vi "Autonomous Independent.vi"() -> ()   [LabVIEW 2016]
doc: "This VI is called when autonomous begins, and will automatically be terminated when autonomous ends. You can carry out timed or sensor driven robot movement independently without needing to return to the caller."
uses:
  <vilib>/Rock Robotics/WPI/Solenoid/WPI_SolenoidValue.ctl
  <vilib>/Rock Robotics/WPI/Utilities/WPI_GetSetVariantRefNum.vi
  <vilib>/Rock Robotics/Network Tables/NT Write Numeric Array.vi
  <vilib>/Rock Robotics/Network Tables/NT Read String.vi
  <vilib>/Rock Robotics/WPI/RobotDrive/WPI_RobotDriveArcadeDrive_Standard(NoSaturation).vi
  <vilib>/Rock Robotics/WPI/Solenoid/WPI_SolenoidSetEnum.vi
panel:
  out "encodervalue 2":dbl
  out "Current Movement, for debugging":T1 {"Y Joystick Value" scale=1.0..-1.0; "X Joystick Value" scale=-1.0..1.0}
  in  "Array of robot movements":T2(array[cluster])=[{"X Joystick Value"=0.39393939393939403, "Y Joystick Value"=0.0, "Delay (sec)"=1.0, "Movement Name"="turn"}, {"X Joystick Value"=-0.3737373737373737, "Y Joystick Value"=0.0, "Delay (sec)"=1.0, "Movement Name"="turn back"}] {"Y Joystick Value" scale=1.0..-1.0; "X Joystick Value" scale=-1.0..1.0}
  out "encodervalue":dbl
  # "Be sure to right-click and choose Data Operations>>Make Current Value default if you want to save the array values with the VI"
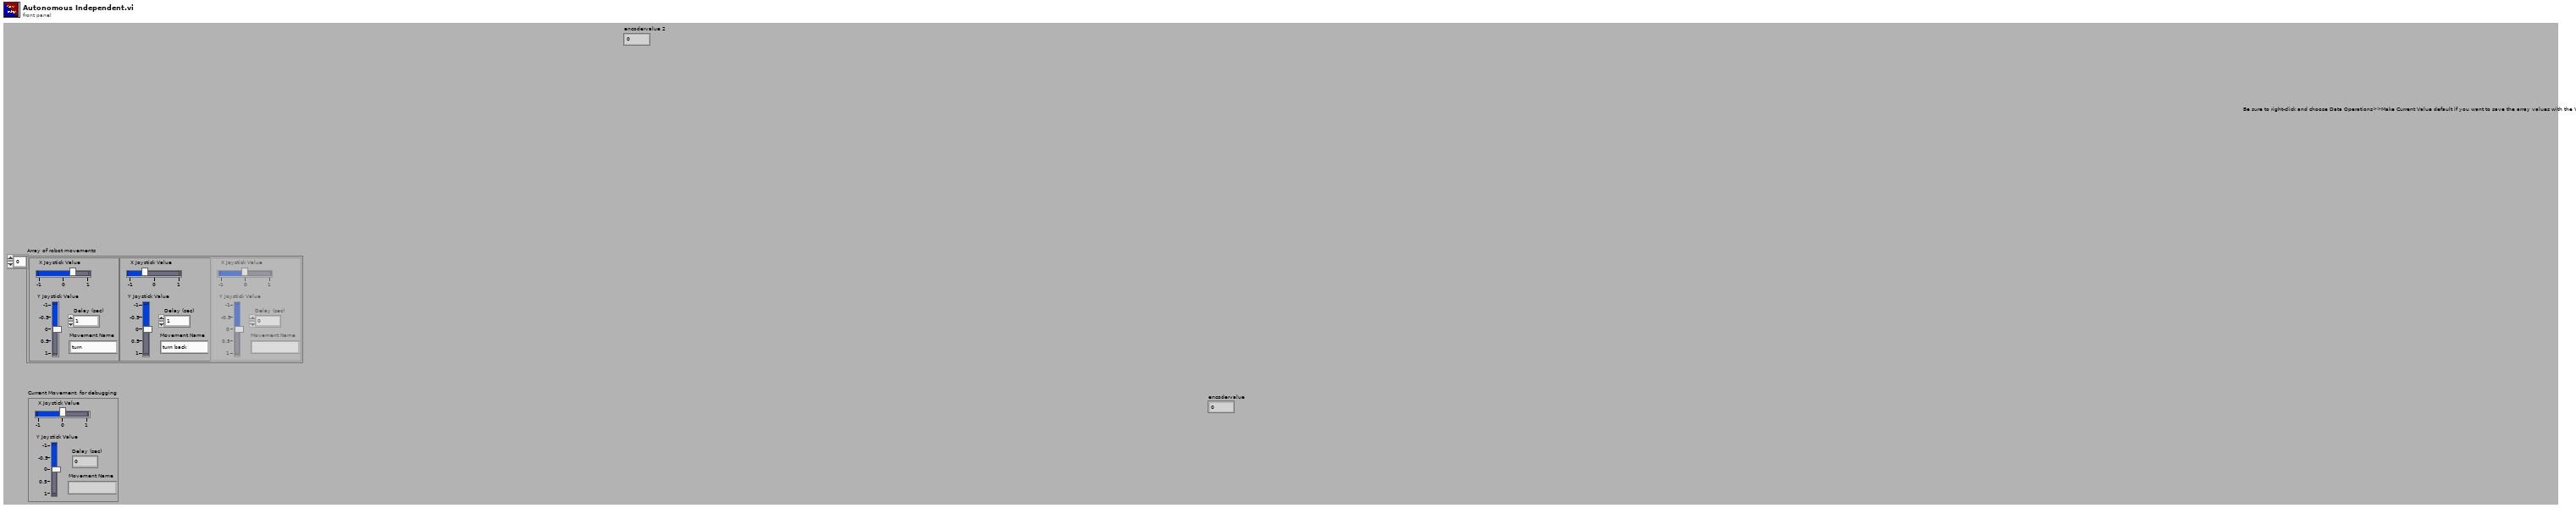
[diagram p1: front panel]
types:
  T1 = cluster{"X Joystick Value":dbl, "Y Joystick Value":dbl, "Delay (sec)":dbl, "Movement Name":string}
  T2 = cluster{"X Joystick Value":dbl, "Y Joystick Value":dbl, "Delay (sec)":dbl, "Movement Name":string}[]
  T3 = typedef "WPI_JoystickDevRef.ctl" = cluster{"Device":T4}
  T4 = typedef "WPI_JoystickDeviceEnum.ctl" = enum16{"USB 0", "USB 1", "USB 2", "USB 3", "USB 4", "USB 5"}
  T5 = typedef "WPI_EncoderDevRef.ctl" = cluster{"DevStatus":errorcluster, "EncoderIndex":T6, "CounterIndex":T7, "DistancePerCount":dbl, "Decoding Type":T8}
  T6 = typedef "FPGA_EncoderIdx.ctl" = enum8{"Enc 0", "Enc 1", "Enc 2", "Enc 3", "Enc 4", "Enc 5", "Enc 6", "Enc 7", "Invalid"}
  T7 = typedef "FPGA_CounterCtrSystemIndex.ctl" = enum8{"Ctr 0", "Ctr 1", "Ctr 2", "Ctr 3", "Ctr 4", "Ctr 5", "Ctr 6", "Ctr 7", "Invalid"}
  T8 = typedef "WPI_EncoderType.ctl" = enum16{"1x", "2x", "4x"}
  T9 = typedef "WPI_GyroDevRef.ctl" = cluster{"DevStatus":errorcluster, "Analog Channel":T10, "Offset":dbl, "Gain (VoltsPerDegree/Second)":dbl, "Gyro Type":enum16{"Analog", "XRS450"}, "Handle":i32, "SPI Bus":T11, "Device Found":bool, "Sample Rate":dbl, "Calibrate On Open":bool}
  T10 = typedef "FPGA_AIChannel.ctl" = enum8{"AI 0", "AI 1", "AI 2", "AI 3", "AI MXP 0", "AI MXP 1", "AI MXP 2", "AI MXP 3", "Invalid"}
  T11 = typedef "spi_bus.ctl" = enum16{"SPI On-Board, CS0", "SPI On-Board, CS1", "SPI On-Board, CS2", "SPI On-Board, CS3", "SPI MXP", "Invalid"}
  T12 = typedef "WPI_RobotDriveDevRef.ctl" = cluster{"DevStatus":errorcluster, "Motors[]":T13[], "Square Inputs":bool, "Max Output":dbl}
  T13 = typedef "WPI_MotorControlDeviceRef.ctl" = cluster{"DeviceStatus":errorcluster, "Type":T14, "PWM":cluster{"PWM Channel":T15, "DeadBand":T16}, "CAN":cluster{"Device Number":u8, "SetOutput VI Ref":variant, "GetOutput VI Ref":variant, "Enable VI Ref":variant, "Disable VI Ref":variant, "Data":variant}, "Invert":bool}
  T14 = typedef "WPI_MotorControlType.ctl" = enum16{"PWM", "CAN"}
  T15 = typedef "FPGA_DIOPWMChannel.ctl" = enum8{"PWM 0", "PWM 1", "PWM 2", "PWM 3", "PWM 4", "PWM 5", "PWM 6", "PWM 7", "PWM 8", "PWM 9", "PWM MXP 0", "PWM MXP 1", "PWM MXP 2", "PWM MXP 3", "PWM MXP 4", "PWM MXP 5", "PWM MXP 6", "PWM MXP 7", "PWM MXP 8", "PWM MXP 9", "Invalid"}
  T16 = typedef "WPI_PWMDeadband.ctl" = cluster{"Name":string, "maxPositivePwm":i32, "minPositivePwm":i32, "centerPwm":i32, "maxNegativePwm":i32, "minNegativePwm":i32, "angularRange":u16}
  T17 = typedef "WPI_SolenoidDevRef.ctl" = cluster{"DevStatus":errorcluster, "Pneumatics Control Module":u8, "Forward Solenoid Channel":T18, "Reverse Solenoid Channel":T18}
  T18 = typedef "WPI_SolenoidChannel.ctl" = enum8{"Solenoid 0", "Solenoid 1", "Solenoid 2", "Solenoid 3", "Solenoid 4", "Solenoid 5", "Solenoid 6", "Solenoid 7", "Invalid"}
  T19 = typedef "WPI_SolenoidValue.ctl" = enum16{"Off", "On", "Forward", "Reverse"}
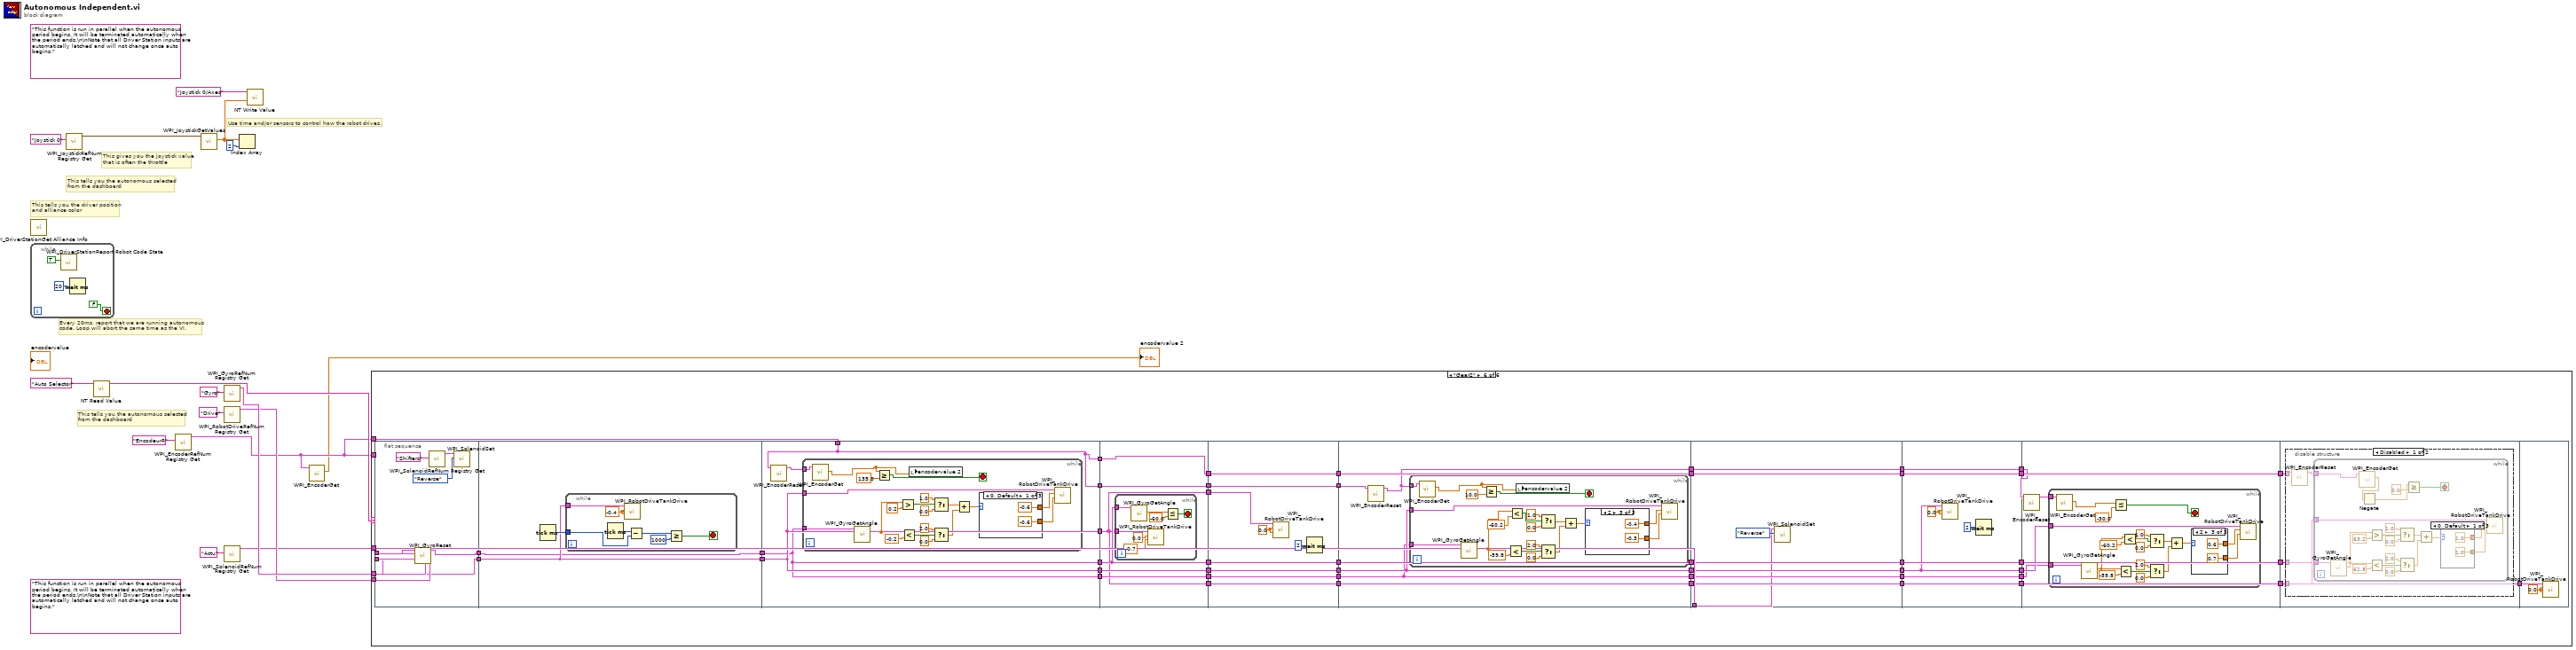
[diagram p0: block diagram]
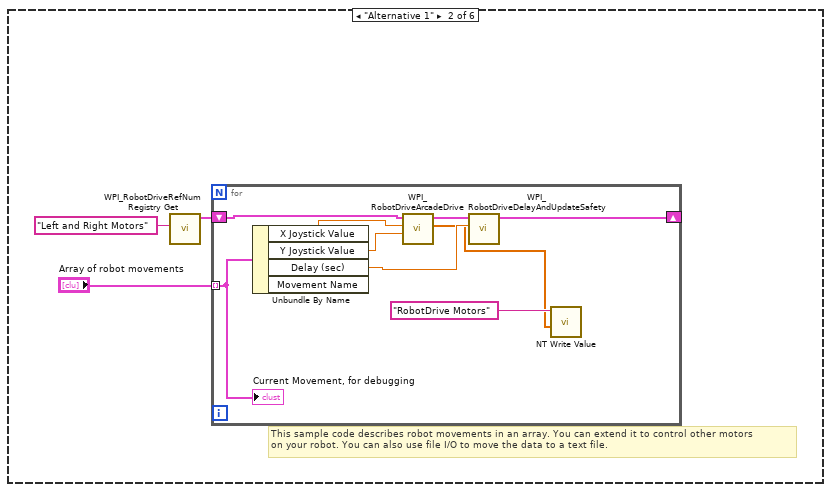
[diagram p3: hidden frame]
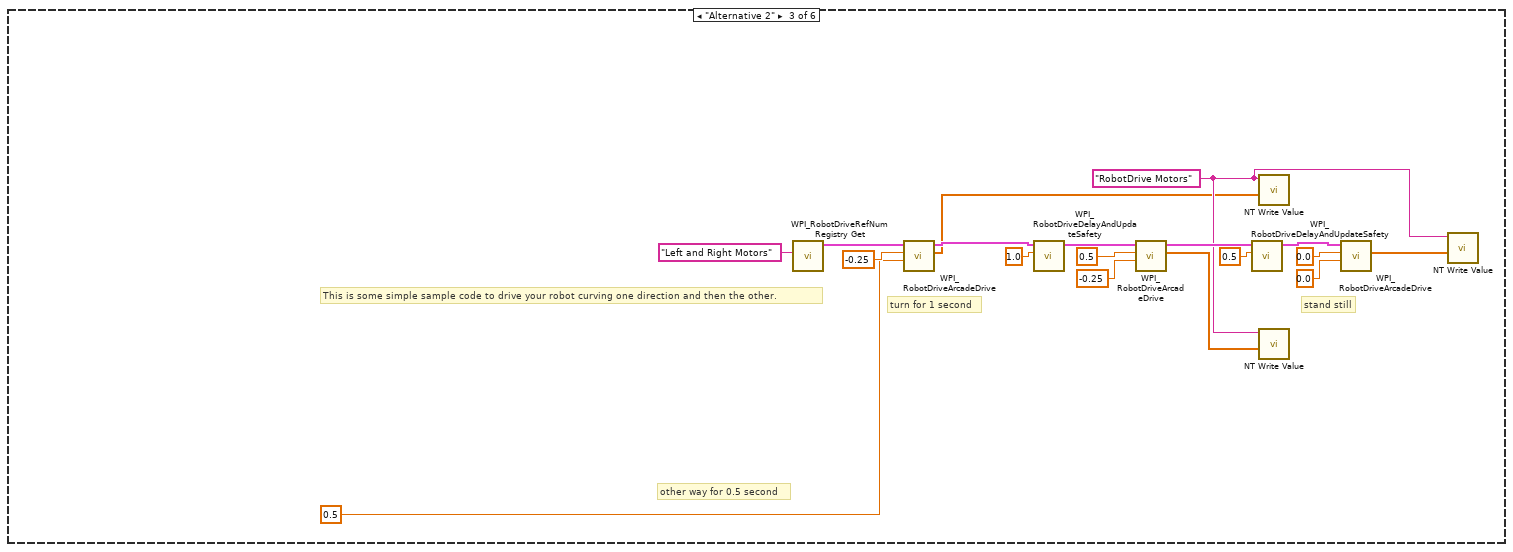
[diagram p4: hidden frame]
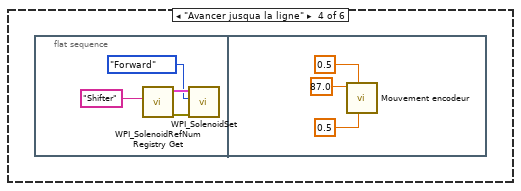
[diagram p5: hidden frame]
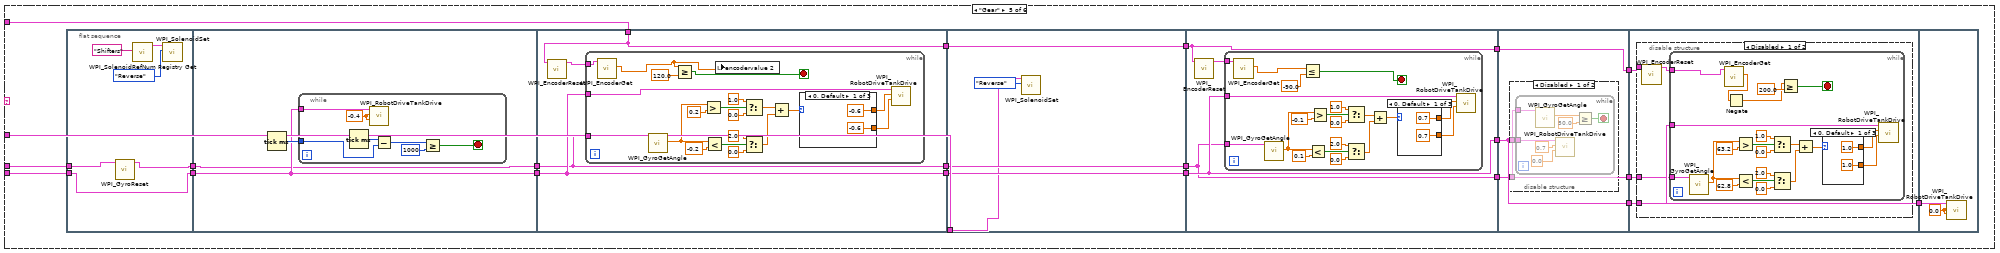
[diagram p6: hidden frame]
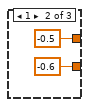
[diagram p7: hidden frame]
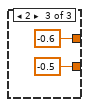
[diagram p8: hidden frame]
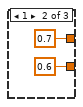
[diagram p9: hidden frame]
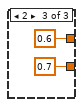
[diagram p10: hidden frame]
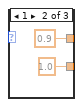
[diagram p12: hidden frame]
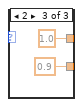
[diagram p13: hidden frame]
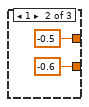
[diagram p15: hidden frame]
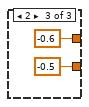
[diagram p16: hidden frame]
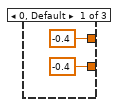
[diagram p17: hidden frame]
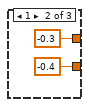
[diagram p18: hidden frame]
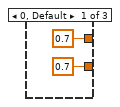
[diagram p19: hidden frame]
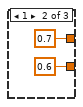
[diagram p20: hidden frame]
diagram:
  (unwired) "This function is run in parallel when the autonomous period begins. It will be terminated automatically when the period ends.\n\nNote that all Driver Station inputs are automatically latched and will not change once auto begins."
  (unwired) "This function is run in parallel when the autonomous period begins. It will be terminated automatically when the period ends.\n\nNote that all Driver Station inputs are automatically latched and will not change once auto begins."
  # "This tells you the autonomous selected\nfrom the dashboard"
  # "This tells you the autonomous selected\nfrom the dashboard"
  # "Every 20ms, report that we are running autonomous\ncode. Loop will abort the same time as the VI."
  # "This gives you the joystick value\nthat is often the throttle"
  # "Use time and/or sensors to control how the robot drives."
  # "This tells you the driver position\nand alliance color"
  n1 = call <vilib>:"WPI_DriverStationGet Alliance Info.vi"() -> ()  [unwired: 12 out]
  n2 = while {
    stop <- FALSE stop-if-true
    n3 = call <vilib>:"WPI_DriverStationReport Robot Code State.vi"("Autonomous"=TRUE) -> ()  [unwired: 10 in, 1 out]
    n4 = Wait (ms)(milliseconds to wait=u32 20) -> ()  [unwired: 1 out]
  }
  n5 = call <vilib>:"WPI_JoystickRefNum Registry Get.vi"("refnum name"="Joystick 0") -> ("JoystickDevRef"=w15:T3)  [unwired: 1 in, 9 out]
  n6 = call-poly <vilib>:"NT Read Value.vi"("Name"="Auto Selector") -> ("String"=w4:string)  [unwired: 9 in, 1 out]
  n7 = call <vilib>:"WPI_EncoderRefNum Registry Get.vi"("refnum name"="EncodeurR") -> ("EncoderDevRef"=w2:T5)  [unwired: 9 in, 1 out]
  n8 = call <vilib>:"WPI_JoystickGetValues.vi"("JoystickDevRef"=w15) -> ("Axes"=w13:dbl[])  [unwired: 6 in, 4 out]
  n9 = call <vilib>:"WPI_GyroRefNum Registry Get.vi"("refnum name"="Gyro") -> ("GyroDevRef"=w6:T9)  [unwired: 9 in, 1 out]
  n10 = call <vilib>:"WPI_RobotDriveRefNum Registry Get.vi"("refnum name"="Drive") -> ("RobotDriveDevRef"=w5:T12)  [unwired: 9 in, 1 out]
  n11 = call <vilib>:"WPI_SolenoidRefNum Registry Get.vi"("refnum name"="Actu") -> ("SolenoidDevRef"=w3:T17)  [unwired: 9 in, 1 out]
  n12 = Index Array(array=w13, index=2) -> ()  [unwired: 1 out]
  n13 = call-poly <vilib>:"NT Write Value.vi"("Numeric Array"=w13, "Name"="Joystick 0/Axes") -> ()  [unwired: 9 in, 1 out]
  n14 = call <vilib>:"WPI_EncoderGet.vi"("EncoderDevRef"=w2) -> ("Distance"=→"encodervalue 2":dbl)  [unwired: 5 in, 5 out]
  n15 = case shown="\"Gear2\"" w4 {
    tunnel: w5 -> [_ _ _ _ w77 w249]
    tunnel: w6 -> [_ _ _ _ w72 w250]
    tunnel: w2 -> [_ _ _ _ w66 _]
    tunnel: w2 -> [_ _ _ _ _ w248]
    tunnel: w3 -> [_ _ _ _ w57 w219]
    frame Default {
      # "You can put your main auto here, or you can right-click on the case and make any\nother frame be the default case."
      # "This is the frame that will execute if no selection is made, or if it is not recognized"
    }
    frame "Alternative 1" {
      # "This sample code describes robot movements in an array. You can extend it to control other motors\non your robot. You can also use file I/O to move the data to a text file."
      n16 = call <vilib>:"WPI_RobotDriveRefNum Registry Get.vi"("refnum name"="Left and Right Motors") -> ("RobotDriveDevRef"=w21:T12)  [unwired: 1 in, 9 out]
      n17 = for {
        shift-right: [w29] -> _
        shift-left: w21 -> [w30]
        tunnel: "Array of robot movements" -> [w25] mode=indexing
        n18 = Unbundle By Name(w25) -> ("X Joystick Value"=w28:dbl, "Y Joystick Value"=w27:dbl, "Delay (sec)"=w26:dbl)  [unwired: 1 out]
        n19 = call-poly <vilib>:"WPI_RobotDriveArcadeDrive.vi"("Y axis value"=w27, "X axis value"=w28, "RobotDriveDevRef"=w30) -> ("Motor Values"=w23:dbl[], "RobotDriveDevRef"=w31:T12)  [unwired: 1 in, 6 out]
        n20 = call <vilib>:"WPI_RobotDriveDelayAndUpdateSafety.vi"("Delay (s)"=w26, "RobotDriveDevRef"=w31) -> ("RobotDriveDevRef 2"=w29:T12)  [unwired: 8 in, 1 out]
        n21 = call-poly <vilib>:"NT Write Value.vi"("Numeric Array"=w23, "Name"="RobotDrive Motors") -> ()  [unwired: 9 in, 1 out]
        "Current Movement, for debugging" <- w25
      }
    }
    frame "Alternative 2" {
      w33 = "RobotDrive Motors" ("Name")
      # "This is some simple sample code to drive your robot curving one direction and then the other."
      # "stand still"
      # "other way for 0.5 second"
      # "turn for 1 second"
      n22 = call <vilib>:"WPI_RobotDriveRefNum Registry Get.vi"("refnum name"="Left and Right Motors") -> ("RobotDriveDevRef"=w49:T12)  [unwired: 1 in, 9 out]
      n23 = call-poly <vilib>:"WPI_RobotDriveArcadeDrive.vi"("Y axis value"=0.5 ("X axis value"), "X axis value"=-0.25, "RobotDriveDevRef"=w49) -> ("Motor Values"=w32:dbl[], "RobotDriveDevRef"=w42:T12)  [unwired: 1 in, 6 out]
      n24 = call <vilib>:"WPI_RobotDriveDelayAndUpdateSafety.vi"("Delay (s)"=1.0, "RobotDriveDevRef"=w42) -> ("RobotDriveDevRef 2"=w43:T12)  [unwired: 8 in, 1 out]
      n25 = call-poly <vilib>:"WPI_RobotDriveArcadeDrive.vi"("Y axis value"=-0.25 ("X axis value"), "X axis value"=0.5, "RobotDriveDevRef"=w43) -> ("Motor Values"=w34:dbl[], "RobotDriveDevRef"=w44:T12)  [unwired: 1 in, 6 out]
      n26 = call <vilib>:"WPI_RobotDriveDelayAndUpdateSafety.vi"("Delay (s)"=0.5, "RobotDriveDevRef"=w44) -> ("RobotDriveDevRef 2"=w45:T12)  [unwired: 8 in, 1 out]
      n27 = call-poly <vilib>:"NT Write Value.vi"("Numeric Array"=w32, "Name"=w33) -> ()  [unwired: 9 in, 1 out]
      n28 = call-poly <vilib>:"NT Write Value.vi"("Numeric Array"=w34, "Name"=w33) -> ()  [unwired: 9 in, 1 out]
      n29 = call-poly <vilib>:"WPI_RobotDriveArcadeDrive.vi"("Y axis value"=0.0 ("X axis value"), "X axis value"=0.0, "RobotDriveDevRef"=w45) -> ("Motor Values"=w35:dbl[])  [unwired: 1 in, 7 out]
      n30 = call-poly <vilib>:"NT Write Value.vi"("Numeric Array"=w35, "Name"=w33) -> ()  [unwired: 9 in, 1 out]
    }
    frame "Avancer jusqua la ligne" {
      n31 = flat-sequence {
        frame #0 {
          n32 = call <vilib>:"WPI_SolenoidRefNum Registry Get.vi"("refnum name"="Shifter") -> ("error out"=w52:errorcluster, "SolenoidDevRef"=w51:T17)  [unwired: 9 in]
          n33 = call-poly <vilib>:"WPI_SolenoidSet.vi"("error in (no error)"=w52, "Value"=WPI_SolenoidValue."Forward", "SolenoidDevRef"=w51) -> ()  [unwired: 7 in, 2 out]
        }
        frame #1 {
          n34 = call "Mouvement encodeur.vi"("Vitesse initiale"=0.5, "Temps acceleration"=0.5, "Distance"=87.0) -> ()  [unwired: 9 in]
        }
      }
    }
    frame "Gear" {
      n35 = flat-sequence {
        tunnel: [w79] -> w76
        tunnel: w77 -> [w79]
        tunnel: [w78] -> w73
        tunnel: w72 -> [w80]
        tunnel: w76 -> [w85]
        tunnel: [w85] -> w75
        tunnel: [w84] -> w74
        tunnel: w73 -> [w84]
        tunnel: w75 -> [w97]
        tunnel: [w97] -> w63
        tunnel: w74 -> [w96]
        tunnel: [w96] -> w61
        tunnel: w66 -> [w95]
        tunnel: [w95] -> w59
        tunnel: w63 -> [w128]
        tunnel: [w128] -> w62
        tunnel: w61 -> [w127]
        tunnel: [w127] -> w60
        tunnel: w59 -> [w126]
        tunnel: [w126] -> w58
        tunnel: w57 -> [w125]
        tunnel: w62 -> [w132]
        tunnel: [w132] -> w71
        tunnel: w60 -> [w131]
        tunnel: [w131] -> w70
        tunnel: w58 -> [w130]
        tunnel: [w130] -> w65
        tunnel: w71 -> [w161]
        tunnel: [w161] -> w69
        tunnel: w70 -> [w160]
        tunnel: [w160] -> w67
        tunnel: w65 -> [w159]
        tunnel: [w159] -> w64
        tunnel: w69 -> [w173]
        tunnel: [w173] -> w68
        tunnel: w67 -> [w172]
        tunnel: w64 -> [w171]
        tunnel: w68 -> [w205]
        frame #0 {
          n36 = call <vilib>:"WPI_GyroReset.vi"("GyroDevRef"=w80) -> ("GyroDevRef"=w78:T9)  [unwired: 9 in, 1 out]
          n37 = call <vilib>:"WPI_SolenoidRefNum Registry Get.vi"("refnum name"="Shifters") -> ("SolenoidDevRef"=w83:T17)  [unwired: 9 in, 1 out]
          n38 = call-poly <vilib>:"WPI_SolenoidSet.vi"("Value"=WPI_SolenoidValue."Reverse", "SolenoidDevRef"=w83) -> ()  [unwired: 8 in, 2 out]
        }
        frame #1 {
          n39 = Tick Count (ms)() -> (millisecond timer value=w86:u32)
          n40 = while {
            tunnel: w85 -> [w92]
            tunnel: w86 -> [w90]
            stop <- w87 stop-if-true
            w93 = -0.4 ("Left axis value")
            n41 = Tick Count (ms)() -> (millisecond timer value=w91:u32)
            n42 = call <vilib>:"WPI_RobotDriveTankDrive.vi"("Right axis value"=w93, "Left axis value"=w93, "RobotDriveDevRef"=w92) -> ()  [unwired: 6 in, 3 out]
            n43 = Subtract(x=w91, y=w90) -> (x-y=w89:u32)
            n44 = Greater Or Equal?(x=w89, y=u32 1000) -> (x >= y?=w87:bool)
          }
        }
        frame #2 {
          n45 = call <vilib>:"WPI_EncoderReset.vi"("EncoderDevRef"=w95) -> ("EncoderDevRef"=w94:T5)  [unwired: 9 in, 1 out]
          n46 = while {
            tunnel: w97 -> [w117]
            tunnel: w96 -> [w116]
            tunnel: w94 -> [w99]
            stop <- w100 stop-if-true
            n47 = call <vilib>:"WPI_EncoderGet.vi"("EncoderDevRef"=w99) -> ("Distance"=w98:dbl)  [unwired: 5 in, 5 out]
            n48 = call <vilib>:"WPI_GyroGetAngle.vi"("GyroDevRef"=w116) -> ("Angle"=w103:dbl)  [unwired: 6 in, 4 out]
            n49 = Greater Or Equal?(x=w98, y=120.0) -> (x >= y?=w100:bool)
            n50 = Greater?(x=w103, y=0.2) -> (0:w114:bool)
            n51 = Less?(x=w103, y=-0.2) -> (x < y?=w102:bool)
            n52 = local write "encodervalue 2"(w98) -> ()
            n53 = Select(t=1.0, s=w114, f=0.0) -> (s? t:f=w109:dbl)
            n54 = Select(t=2.0, s=w102, f=0.0) -> (s? t:f=w108:dbl)
            n55 = Add(x=w109, y=w108) -> (x+y=w107:dbl)
            n56 = case shown="0, Default" w107 {
              tunnel: [-0.6 ("t") -0.5 ("t") -0.6 ("t")] -> w106
              tunnel: [-0.6 ("f") -0.6 ("f") -0.5 ("f")] -> w105
              frame 0, Default {
              }
              frame 1 {
              }
              frame 2 {
              }
            }
            n57 = call <vilib>:"WPI_RobotDriveTankDrive.vi"("Right axis value"=w105, "Left axis value"=w106, "RobotDriveDevRef"=w117) -> ()  [unwired: 6 in, 3 out]
          }
        }
        frame #3 {
          n58 = call-poly <vilib>:"WPI_SolenoidSet.vi"("Value"=WPI_SolenoidValue."Reverse", "SolenoidDevRef"=w125) -> ()  [unwired: 8 in, 2 out]
        }
        frame #4 {
          n59 = call <vilib>:"WPI_EncoderReset.vi"("EncoderDevRef"=w130) -> ("EncoderDevRef"=w129:T5)  [unwired: 9 in, 1 out]
          n60 = while {
            tunnel: w132 -> [w140]
            tunnel: w131 -> [w137]
            tunnel: w129 -> [w134]
            stop <- w135 stop-if-true
            n61 = call <vilib>:"WPI_EncoderGet.vi"("EncoderDevRef"=w134) -> ("Distance"=w133:dbl)  [unwired: 5 in, 5 out]
            n62 = call <vilib>:"WPI_GyroGetAngle.vi"("GyroDevRef"=w137) -> ("Angle"=w151:dbl)  [unwired: 6 in, 4 out]
            n63 = Less Or Equal?(x=w133, y=-90.0) -> (x <= y?=w135:bool)
            n64 = Less?(x=w151, y=0.1) -> (x < y?=w152:bool)
            n65 = Greater?(x=w151, y=-0.1) -> (0:w142:bool)
            n66 = Select(t=1.0, s=w142, f=0.0) -> (s? t:f=w147:dbl)
            n67 = Select(t=2.0, s=w152, f=0.0) -> (s? t:f=w148:dbl)
            n68 = Add(x=w147, y=w148) -> (x+y=w149:dbl)
            n69 = case shown="0, Default" w149 {
              tunnel: [0.7 ("t") 0.7 ("t") 0.6 ("t")] -> w139
              tunnel: [0.7 ("f") 0.6 ("f") 0.7 ("f")] -> w138
              frame 0, Default {
              }
              frame 1 {
              }
              frame 2 {
              }
            }
            n70 = call <vilib>:"WPI_RobotDriveTankDrive.vi"("Right axis value"=w138, "Left axis value"=w139, "RobotDriveDevRef"=w140) -> ()  [unwired: 6 in, 3 out]
          }
        }
        frame #5 {
          n71 = disable-structure shown="Disabled" {
            disable-tunnel: w161 -> [w163 _]
            disable-tunnel: w160 -> [w162 _]
            frame Disabled {
              n72 = while {
                tunnel: w162 -> [w167]
                tunnel: w163 -> [w164]
                stop <- w168 stop-if-true
                n73 = call <vilib>:"WPI_GyroGetAngle.vi"("GyroDevRef"=w167) -> ("Angle"=w170:dbl)  [unwired: 6 in, 4 out]
                n74 = call <vilib>:"WPI_RobotDriveTankDrive.vi"("Right axis value"=0.0, "Left axis value"=0.7, "RobotDriveDevRef"=w164) -> ()  [unwired: 6 in, 3 out]
                n75 = Greater Or Equal?(x=w170, y=50.0) -> (x >= y?=w168:bool)
              }
            }
            frame Enabled {
            }
          }
        }
        frame #6 {
          n76 = disable-structure shown="Disabled" {
            disable-tunnel: w173 -> [w177 _]
            disable-tunnel: w172 -> [w176 _]
            disable-tunnel: w171 -> [w175 _]
            frame Disabled {
              n77 = call <vilib>:"WPI_EncoderReset.vi"("EncoderDevRef"=w175) -> ("EncoderDevRef"=w174:T5)  [unwired: 9 in, 1 out]
              n78 = while {
                tunnel: w177 -> [w198]
                tunnel: w176 -> [w196]
                tunnel: w174 -> [w180]
                stop <- w197 stop-if-true
                n79 = call <vilib>:"WPI_GyroGetAngle.vi"("GyroDevRef"=w196) -> ("Angle"=w183:dbl)  [unwired: 6 in, 4 out]
                n80 = call <vilib>:"WPI_EncoderGet.vi"("EncoderDevRef"=w180) -> ("Distance"=w179:dbl)  [unwired: 5 in, 5 out]
                n81 = Negate(x=w179) -> (-x=w178:dbl)
                n82 = Greater?(x=w183, y=63.2) -> (0:w194:bool)
                n83 = Less?(x=w183, y=62.8) -> (x < y?=w182:bool)
                n84 = Select(t=1.0, s=w194, f=0.0) -> (s? t:f=w189:dbl)
                n85 = Select(t=2.0, s=w182, f=0.0) -> (s? t:f=w188:dbl)
                n86 = Greater Or Equal?(x=w178, y=200.0) -> (x >= y?=w197:bool)
                n87 = Add(x=w189, y=w188) -> (x+y=w187:dbl)
                n88 = case shown="0, Default" w187 {
                  tunnel: [1.0 ("t") 0.9 ("t") 1.0 ("t")] -> w186
                  tunnel: [1.0 ("f") 1.0 ("f") 0.9 ("f")] -> w185
                  frame 0, Default {
                  }
                  frame 1 {
                  }
                  frame 2 {
                  }
                }
                n89 = call <vilib>:"WPI_RobotDriveTankDrive.vi"("Right axis value"=w185, "Left axis value"=w186, "RobotDriveDevRef"=w198) -> ()  [unwired: 6 in, 3 out]
              }
            }
            frame Enabled {
            }
          }
        }
        frame #7 {
          w206 = 0.0 ("Left axis value")
          n90 = call <vilib>:"WPI_RobotDriveTankDrive.vi"("Right axis value"=w206, "Left axis value"=w206, "RobotDriveDevRef"=w205) -> ()  [unwired: 6 in, 3 out]
        }
      }
    }
    frame "Gear2" {
      n91 = flat-sequence {
        tunnel: [w257] -> w255
        tunnel: w249 -> [w257]
        tunnel: [w256] -> w254
        tunnel: w250 -> [w258]
        tunnel: w255 -> [w263]
        tunnel: [w263] -> w253
        tunnel: [w262] -> w252
        tunnel: w254 -> [w262]
        tunnel: w253 -> [w274]
        tunnel: [w274] -> w247
        tunnel: w252 -> [w273]
        tunnel: [w273] -> w246
        tunnel: w248 -> [w272]
        tunnel: [w272] -> w245
        tunnel: [w274] -> w244
        tunnel: [w273] -> w243
        tunnel: [w272] -> w242
        tunnel: w247 -> [w302]
        tunnel: [w302] -> w238
        tunnel: w246 -> [w307]
        tunnel: [w307] -> w236
        tunnel: [w306] -> w234
        tunnel: w245 -> [w306]
        tunnel: [w305] -> w232
        tunnel: w244 -> [w305]
        tunnel: [w304] -> w230
        tunnel: w243 -> [w304]
        tunnel: [w303] -> w228
        tunnel: w242 -> [w303]
        tunnel: [w302] -> w226
        tunnel: w238 -> [w323]
        tunnel: [w323] -> w237
        tunnel: w236 -> [w322]
        tunnel: [w322] -> w235
        tunnel: w234 -> [w321]
        tunnel: [w321] -> w233
        tunnel: w232 -> [w320]
        tunnel: [w320] -> w231
        tunnel: w230 -> [w319]
        tunnel: [w319] -> w229
        tunnel: w228 -> [w318]
        tunnel: [w318] -> w227
        tunnel: w226 -> [w316]
        tunnel: w237 -> [w330]
        tunnel: [w330] -> w225
        tunnel: w235 -> [w329]
        tunnel: [w329] -> w224
        tunnel: w233 -> [w328]
        tunnel: [w328] -> w223
        tunnel: w231 -> [w327]
        tunnel: w229 -> [w326]
        tunnel: w227 -> [w324]
        tunnel: [w327] -> w222
        tunnel: [w326] -> w221
        tunnel: [w325] -> w220
        tunnel: w225 -> [w364]
        tunnel: [w364] -> w218
        tunnel: w224 -> [w363]
        tunnel: [w363] -> w216
        tunnel: w223 -> [w362]
        tunnel: [w362] -> w214
        tunnel: w222 -> [w361]
        tunnel: [w361] -> w212
        tunnel: w221 -> [w360]
        tunnel: [w360] -> w210
        tunnel: w220 -> [w359]
        tunnel: [w359] -> w208
        tunnel: w219 -> [w357]
        tunnel: w218 -> [w372]
        tunnel: [w372] -> w217
        tunnel: w216 -> [w371]
        tunnel: [w371] -> w215
        tunnel: w214 -> [w370]
        tunnel: [w370] -> w213
        tunnel: w212 -> [w365]
        tunnel: [w365] -> w211
        tunnel: w210 -> [w369]
        tunnel: [w369] -> w209
        tunnel: w208 -> [w368]
        tunnel: [w368] -> w207
        tunnel: w217 -> [w379]
        tunnel: [w379] -> w241
        tunnel: w215 -> [w378]
        tunnel: [w378] -> w240
        tunnel: w213 -> [w377]
        tunnel: [w377] -> w239
        tunnel: w211 -> [w375]
        tunnel: w209 -> [w374]
        tunnel: w207 -> [w373]
        tunnel: w241 -> [w408]
        tunnel: [w408] -> w251
        tunnel: w240 -> [w407]
        tunnel: w239 -> [w406]
        tunnel: w251 -> [w440]
        frame #0 {
          n92 = call <vilib>:"WPI_GyroReset.vi"("GyroDevRef"=w258) -> ("GyroDevRef"=w256:T9)  [unwired: 9 in, 1 out]
          n93 = call <vilib>:"WPI_SolenoidRefNum Registry Get.vi"("refnum name"="Shifters") -> ("SolenoidDevRef"=w261:T17)  [unwired: 9 in, 1 out]
          n94 = call-poly <vilib>:"WPI_SolenoidSet.vi"("Value"=WPI_SolenoidValue."Reverse", "SolenoidDevRef"=w261) -> ()  [unwired: 8 in, 2 out]
        }
        frame #1 {
          n95 = Tick Count (ms)() -> (millisecond timer value=w264:u32)
          n96 = while {
            tunnel: w263 -> [w270]
            tunnel: w264 -> [w268]
            stop <- w265 stop-if-true
            w271 = -0.4 ("Left axis value")
            n97 = Tick Count (ms)() -> (millisecond timer value=w269:u32)
            n98 = call <vilib>:"WPI_RobotDriveTankDrive.vi"("Right axis value"=w271, "Left axis value"=w271, "RobotDriveDevRef"=w270) -> ()  [unwired: 6 in, 3 out]
            n99 = Subtract(x=w269, y=w268) -> (x-y=w267:u32)
            n100 = Greater Or Equal?(x=w267, y=u32 1000) -> (x >= y?=w265:bool)
          }
        }
        frame #2 {
          n101 = call <vilib>:"WPI_EncoderReset.vi"("EncoderDevRef"=w272) -> ("EncoderDevRef"=w275:T5)  [unwired: 9 in, 1 out]
          n102 = while {
            tunnel: w274 -> [w295]
            tunnel: w273 -> [w294]
            tunnel: w275 -> [w277]
            stop <- w278 stop-if-true
            n103 = call <vilib>:"WPI_EncoderGet.vi"("EncoderDevRef"=w277) -> ("Distance"=w276:dbl)  [unwired: 5 in, 5 out]
            n104 = call <vilib>:"WPI_GyroGetAngle.vi"("GyroDevRef"=w294) -> ("Angle"=w281:dbl)  [unwired: 6 in, 4 out]
            n105 = Greater Or Equal?(x=w276, y=135.0) -> (x >= y?=w278:bool)
            n106 = Greater?(x=w281, y=0.2) -> (0:w292:bool)
            n107 = Less?(x=w281, y=-0.2) -> (x < y?=w280:bool)
            n108 = local write "encodervalue 2"(w276) -> ()
            n109 = Select(t=1.0, s=w292, f=0.0) -> (s? t:f=w287:dbl)
            n110 = Select(t=2.0, s=w280, f=0.0) -> (s? t:f=w286:dbl)
            n111 = Add(x=w287, y=w286) -> (x+y=w285:dbl)
            n112 = case shown="0, Default" w285 {
              tunnel: [-0.6 ("t") -0.5 ("t") -0.6 ("t")] -> w284
              tunnel: [-0.6 ("f") -0.6 ("f") -0.5 ("f")] -> w283
              frame 0, Default {
              }
              frame 1 {
              }
              frame 2 {
              }
            }
            n113 = call <vilib>:"WPI_RobotDriveTankDrive.vi"("Right axis value"=w283, "Left axis value"=w284, "RobotDriveDevRef"=w295) -> ()  [unwired: 6 in, 3 out]
          }
        }
        frame #3 {
          n114 = while {
            tunnel: w307 -> [w311]
            tunnel: w302 -> [w308]
            stop <- w312 stop-if-true
            n115 = call <vilib>:"WPI_GyroGetAngle.vi"("GyroDevRef"=w311) -> ("Angle"=w314:dbl)  [unwired: 6 in, 4 out]
            n116 = call <vilib>:"WPI_RobotDriveTankDrive.vi"("Right axis value"=-0.7, "Left axis value"=0.0, "RobotDriveDevRef"=w308) -> ()  [unwired: 6 in, 3 out]
            n117 = Less Or Equal?(x=w314, y=-60.0) -> (x <= y?=w312:bool)
          }
        }
        frame #4 {
          w317 = 0.0 ("Left axis value")
          n118 = call <vilib>:"WPI_RobotDriveTankDrive.vi"("Right axis value"=w317, "Left axis value"=w317, "RobotDriveDevRef"=w316) -> ()  [unwired: 6 in, 3 out]
          n119 = Wait (ms)(milliseconds to wait=u32 2) -> ()  [unwired: 1 out]
        }
        frame #5 {
          n120 = call <vilib>:"WPI_EncoderReset.vi"("EncoderDevRef"=w324) -> ("EncoderDevRef"=w325:T5)  [unwired: 9 in, 1 out]
          n121 = while {
            tunnel: w327 -> [w350]
            tunnel: w326 -> [w349]
            tunnel: w325 -> [w335]
            stop <- w336 stop-if-true
            n122 = call <vilib>:"WPI_EncoderGet.vi"("EncoderDevRef"=w335) -> ("Distance"=w334:dbl)  [unwired: 5 in, 5 out]
            n123 = call <vilib>:"WPI_GyroGetAngle.vi"("GyroDevRef"=w349) -> ("Angle"=w332:dbl)  [unwired: 6 in, 4 out]
            n124 = Greater Or Equal?(x=w334, y=10.0) -> (x >= y?=w336:bool)
            n125 = Less?(x=w332, y=-59.8) -> (x < y?=w338:bool)
            n126 = Less?(x=w332, y=-60.2) -> (x < y?=w331:bool)
            n127 = local write "encodervalue 2"(w334) -> ()
            n128 = Select(t=1.0, s=w331, f=0.0) -> (s? t:f=w344:dbl)
            n129 = Select(t=2.0, s=w338, f=0.0) -> (s? t:f=w343:dbl)
            n130 = Add(x=w344, y=w343) -> (x+y=w342:dbl)
            n131 = case shown="2" w342 {
              tunnel: [-0.4 ("t") -0.3 ("t") -0.4 ("t")] -> w341
              tunnel: [-0.4 ("f") -0.4 ("f") -0.3 ("f")] -> w340
              frame 0, Default {
              }
              frame 1 {
              }
              frame 2 {
              }
            }
            n132 = call <vilib>:"WPI_RobotDriveTankDrive.vi"("Right axis value"=w340, "Left axis value"=w341, "RobotDriveDevRef"=w350) -> ()  [unwired: 6 in, 3 out]
          }
        }
        frame #6 {
          n133 = call-poly <vilib>:"WPI_SolenoidSet.vi"("Value"=WPI_SolenoidValue."Reverse", "SolenoidDevRef"=w357) -> ()  [unwired: 8 in, 2 out]
        }
        frame #7 {
          w367 = 0.0 ("Left axis value")
          n134 = call <vilib>:"WPI_RobotDriveTankDrive.vi"("Right axis value"=w367, "Left axis value"=w367, "RobotDriveDevRef"=w365) -> ()  [unwired: 6 in, 3 out]
          n135 = Wait (ms)(milliseconds to wait=u32 2) -> ()  [unwired: 1 out]
        }
        frame #8 {
          n136 = call <vilib>:"WPI_EncoderReset.vi"("EncoderDevRef"=w373) -> ("EncoderDevRef"=w376:T5)  [unwired: 9 in, 1 out]
          n137 = while {
            tunnel: w375 -> [w390]
            tunnel: w374 -> [w387]
            tunnel: w376 -> [w384]
            stop <- w385 stop-if-true
            n138 = call <vilib>:"WPI_EncoderGet.vi"("EncoderDevRef"=w384) -> ("Distance"=w383:dbl)  [unwired: 5 in, 5 out]
            n139 = call <vilib>:"WPI_GyroGetAngle.vi"("GyroDevRef"=w387) -> ("Angle"=w381:dbl)  [unwired: 6 in, 4 out]
            n140 = Less Or Equal?(x=w383, y=-30.0) -> (x <= y?=w385:bool)
            n141 = Less?(x=w381, y=-59.8) -> (x < y?=w399:bool)
            n142 = Less?(x=w381, y=-60.2) -> (x < y?=w380:bool)
            n143 = Select(t=1.0, s=w380, f=0.0) -> (s? t:f=w395:dbl)
            n144 = Select(t=2.0, s=w399, f=0.0) -> (s? t:f=w396:dbl)
            n145 = Add(x=w395, y=w396) -> (x+y=w397:dbl)
            n146 = case shown="2" w397 {
              tunnel: [0.7 ("t") 0.7 ("t") 0.6 ("t")] -> w389
              tunnel: [0.7 ("f") 0.6 ("f") 0.7 ("f")] -> w388
              frame 0, Default {
              }
              frame 1 {
              }
              frame 2 {
              }
            }
            n147 = call <vilib>:"WPI_RobotDriveTankDrive.vi"("Right axis value"=w388, "Left axis value"=w389, "RobotDriveDevRef"=w390) -> ()  [unwired: 6 in, 3 out]
          }
        }
        frame #9 {
          n148 = disable-structure shown="Disabled" {
            disable-tunnel: w408 -> [w412 _]
            disable-tunnel: w407 -> [w411 _]
            disable-tunnel: w406 -> [w410 _]
            frame Disabled {
              n149 = call <vilib>:"WPI_EncoderReset.vi"("EncoderDevRef"=w410) -> ("EncoderDevRef"=w409:T5)  [unwired: 9 in, 1 out]
              n150 = while {
                tunnel: w412 -> [w433]
                tunnel: w411 -> [w431]
                tunnel: w409 -> [w415]
                stop <- w432 stop-if-true
                n151 = call <vilib>:"WPI_GyroGetAngle.vi"("GyroDevRef"=w431) -> ("Angle"=w418:dbl)  [unwired: 6 in, 4 out]
                n152 = call <vilib>:"WPI_EncoderGet.vi"("EncoderDevRef"=w415) -> ("Distance"=w414:dbl)  [unwired: 5 in, 5 out]
                n153 = Negate(x=w414) -> (-x=w413:dbl)
                n154 = Greater?(x=w418, y=63.2) -> (0:w429:bool)
                n155 = Less?(x=w418, y=62.8) -> (x < y?=w417:bool)
                n156 = Select(t=1.0, s=w429, f=0.0) -> (s? t:f=w424:dbl)
                n157 = Select(t=2.0, s=w417, f=0.0) -> (s? t:f=w423:dbl)
                n158 = Greater Or Equal?(x=w413, y=0.0) -> (x >= y?=w432:bool)
                n159 = Add(x=w424, y=w423) -> (x+y=w422:dbl)
                n160 = case shown="0, Default" w422 {
                  tunnel: [1.0 ("t") 0.9 ("t") 1.0 ("t")] -> w421
                  tunnel: [1.0 ("f") 1.0 ("f") 0.9 ("f")] -> w420
                  frame 0, Default {
                  }
                  frame 1 {
                  }
                  frame 2 {
                  }
                }
                n161 = call <vilib>:"WPI_RobotDriveTankDrive.vi"("Right axis value"=w420, "Left axis value"=w421, "RobotDriveDevRef"=w433) -> ()  [unwired: 6 in, 3 out]
              }
            }
            frame Enabled {
            }
          }
        }
        frame #10 {
          w441 = 0.0 ("Left axis value")
          n162 = call <vilib>:"WPI_RobotDriveTankDrive.vi"("Right axis value"=w441, "Left axis value"=w441, "RobotDriveDevRef"=w440) -> ()  [unwired: 6 in, 3 out]
        }
      }
    }
  }
